vi "Write Channel.vi"(8 "error in (no error)":errorcluster, 10 "Channel":i32, 11 "Motor-GWInstek in":refnum<class "Motor-GWInstek.lvclass">) -> (0 "error out":errorcluster, 3 "Motor-GWInstek out":refnum<class "Motor-GWInstek.lvclass">)   [LabVIEW 2013, in "PowderDeposition.lvlib" / "Motor-GWInstek.lvclass"]
uses:
  Motor-GWInstek.lvclass
  Motor-GWInstek.lvclass/Motor-GWInstek.ctl
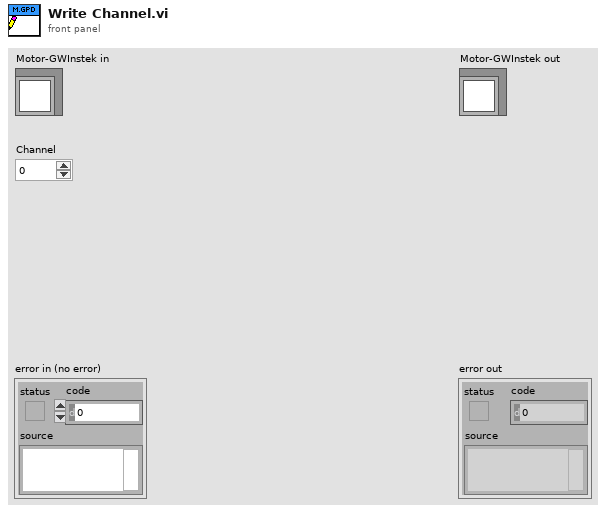
[diagram p1: front panel]
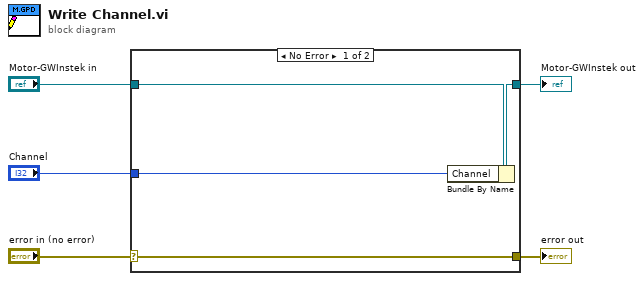
[diagram p0: block diagram]
diagram:
  n1 = case shown="No Error" "error in (no error)" {
    selector: "error in (no error)" -> [w9 w10]
    tunnel: [w9 w10] -> w4
    tunnel: [w7 w11] -> w2
    tunnel: "Motor-GWInstek in" -> [w8 w11]
    tunnel: "Channel" -> [w6 _]
    frame No Error {
      n2 = Bundle By Name(cluster=w8, "Channel"=w6) -> (w7:refnum<class "Motor-GWInstek.lvclass">)
    }
    frame Error {
    }
  }
  "error out" <- w4
  "Motor-GWInstek out" <- w2
